vi "MyFPGA Encoder Counter.vi"(8 "Clear Overflow?":bool, 9 "Signal":bool, 10 "Backward?":bool, 11 "Reset?":bool) -> (1 "Crossed Halfway?":bool, 2 "Wrapped around?":bool, 3 "Count Value":u32, 4 "Crossed Halfway twice?":bool, 5 "Wrapped around twice?":bool)   [LabVIEW 2019]
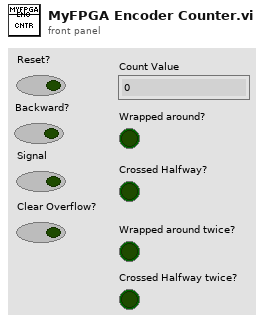
[diagram p1: front panel]
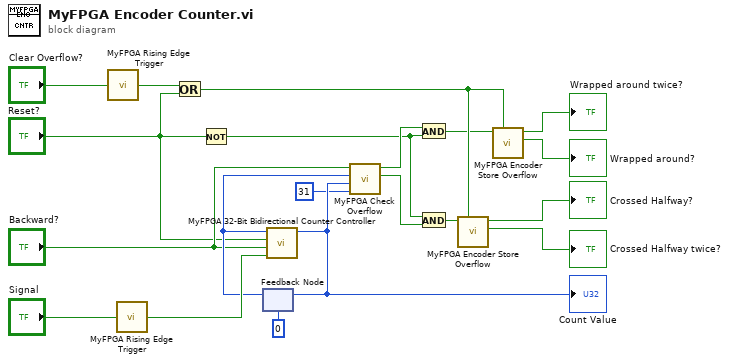
[diagram p0: block diagram]
diagram:
  n1 = call "MyFPGA Rising Edge Trigger.vi"("Signal"="Clear Overflow?") -> ("Trigger?"=w12:bool)
  n2 = call "MyFPGA Rising Edge Trigger.vi"("Signal"="Signal") -> ("Trigger?"=w17:bool)
  n3 = Or(x=w12, y="Reset?") -> (x .or. y?=w9:bool)
  n4 = Not(x="Reset?") -> (.not. x?=w1:bool)
  n5 = feedback #1(u32 0 ("Count Value")) -> (w16:u32)
  n6 = call "MyFPGA 32-Bit Bidirectional Counter Controller.vi"("Enable"=w17, "Direction"="Backward?", "Reset"="Reset?", "Value"=w16) -> ("Value+"=w15:u32)  [unwired: 7 in]
  "Count Value" <- w15
  n7 = feedback-in #1(w15) -> ()
  n8 = call "MyFPGA Check Overflow.vi"("Bit"=u8 31 ("index"), "Current Value"=w15, "Previous Value"=w16, "Backward?"="Backward?") -> ("Crossed Halfway?"=w6:bool, "Wrapped?"=w4:bool)  [unwired: 6 in]
  n9 = And(x=w4, y=w1) -> (x .and. y?=w3:bool)
  n10 = And(x=w1, y=w6) -> (x .and. y?=w5:bool)
  n11 = call "MyFPGA Encoder Store Overflow.vi"("Clear?"=w9, "Over?"=w5) -> ("Error?"=→"Crossed Halfway twice?":bool, "Overflow?"=→"Crossed Halfway?":bool)  [unwired: 8 in]
  n12 = call "MyFPGA Encoder Store Overflow.vi"("Clear?"=w9, "Over?"=w3) -> ("Error?"=→"Wrapped around?":bool, "Overflow?"=→"Wrapped around twice?":bool)  [unwired: 8 in]
